vi "I-V扫描.vi"(0 "VISA资源名称":refnum<visa-resource-name>, 1 "nplc":dbl, 3 "时间点(ms)":dbl, 5 "扫描电压(V)":dbl, 9 "电压改变量":dbl, 11 "错误输入":errorcluster, 12 "极限电流(mA)":dbl, 13 "时序优先":bool, 14 "4-wire":bool) -> (4 "VISA资源名称输出":refnum<visa-resource-name>, 6 "扫描数据":dbl[][](array[numeric]), 10 "时间标识":timestamp, 15 "错误输出":errorcluster)   [LabVIEW 2019]
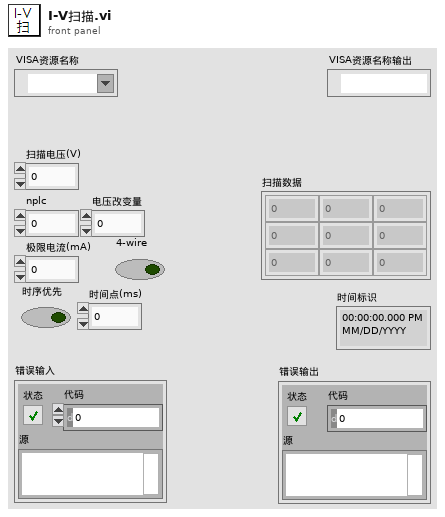
[diagram p1: front panel]
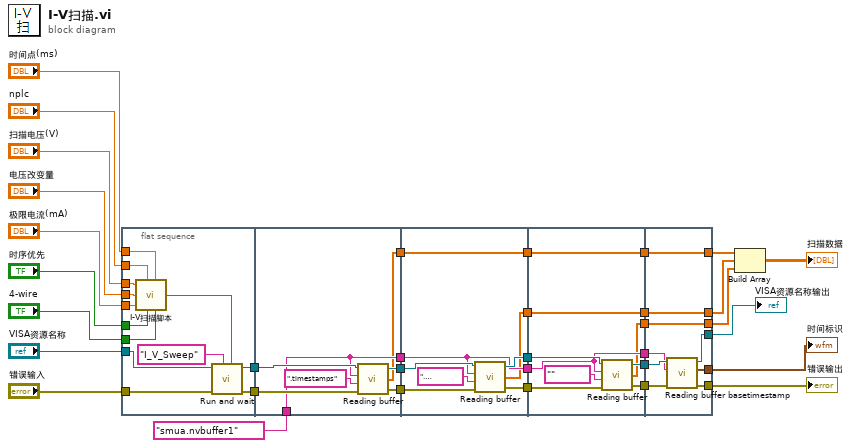
[diagram p0: block diagram]
diagram:
  n1 = flat-sequence {
    tunnel: "错误输入" -> [w46]
    tunnel: "VISA资源名称" -> [w45]
    tunnel: [w44] -> w34
    tunnel: [w43] -> w33
    tunnel: "时间点(ms)" -> [w41]
    tunnel: "时序优先" -> [w40]
    tunnel: "极限电流(mA)" -> [w39]
    tunnel: "电压改变量" -> [w38]
    tunnel: "nplc" -> [w37]
    tunnel: "扫描电压(V)" -> [w36]
    tunnel: "4-wire" -> [w35]
    tunnel: w34 -> [w53]
    tunnel: w33 -> [w52]
    tunnel: [w51] -> w32
    tunnel: [w50] -> w31
    tunnel: [w49] -> w30
    tunnel: "smua.nvbuffer1" ("缓冲区名称") -> [w49]
    tunnel: [w48] -> w29
    tunnel: w32 -> [w61]
    tunnel: w31 -> [w60]
    tunnel: [w59] -> w28
    tunnel: [w58] -> w27
    tunnel: w30 -> [w57]
    tunnel: [w57] -> w26
    tunnel: w29 -> [w56]
    tunnel: [w56] -> w25
    tunnel: [w55] -> w24
    tunnel: w28 -> [w70]
    tunnel: w27 -> [w69]
    tunnel: [w68] -> w23
    tunnel: [w67] -> w22
    tunnel: w26 -> [w66]
    tunnel: [w66] -> w21
    tunnel: w25 -> [w65]
    tunnel: [w65] -> w20
    tunnel: w24 -> [w64]
    tunnel: [w64] -> w19
    tunnel: [w63] -> w18
    tunnel: [w78] -> w14
    tunnel: [w77] -> w15
    tunnel: w23 -> [w80]
    tunnel: w22 -> [w79]
    tunnel: w21 -> [w76]
    tunnel: [w75] -> w12
    tunnel: [w74] -> w10
    tunnel: w20 -> [w74]
    tunnel: w19 -> [w73]
    tunnel: [w73] -> w9
    tunnel: w18 -> [w72]
    tunnel: [w72] -> w8
    frame #0 {
      n2 = call "I-V扫描脚本.vi"("扫描电压(V)"=w36, "nplc"=w37, "电压改变量"=w38, "极限电流(mA)"=w39, "时序优先"=w40, "时间点(ms)"=w41, "4-wire"=w35) -> ("Script"=w42:string)  [unwired: 2 in]
      n3 = call "Run and wait.vi"("Script"=w42, "Script Name"="I_V_Sweep", "错误输入"=w46, "VISA资源名称"=w45) -> ("错误输出"=w44:errorcluster, "VISA资源名称输出"=w43:refnum<visa-resource-name>)  [unwired: 6 in]
    }
    frame #1 {
      n4 = call "Reading buffer.vi"("错误输入"=w53, "Options"=".timestamps", "缓冲区名称"=w49, "VISA资源名称"=w52) -> ("错误输出"=w50:errorcluster, "缓冲区数据"=w48:dbl[], "VISA资源名称输出"=w51:refnum<visa-resource-name>)
    }
    frame #2 {
      n5 = call "Reading buffer.vi"("错误输入"=w60, "Options"=".sourcevalues", "缓冲区名称"=w57, "VISA资源名称"=w61) -> ("错误输出"=w59:errorcluster, "缓冲区数据"=w55:dbl[], "VISA资源名称输出"=w58:refnum<visa-resource-name>)
    }
    frame #3 {
      n6 = call "Reading buffer.vi"("错误输入"=w70, "Options"="", "缓冲区名称"=w66, "VISA资源名称"=w69) -> ("错误输出"=w67:errorcluster, "缓冲区数据"=w63:dbl[], "VISA资源名称输出"=w68:refnum<visa-resource-name>)
    }
    frame #4 {
      n7 = call "Reading buffer basetimestamp.vi"("错误输入"=w79, "缓冲区名称"=w76, "VISA资源名称"=w80) -> ("错误输出"=w78:errorcluster, "时间标识"=w75:timestamp, "VISA资源名称输出"=w77:refnum<visa-resource-name>)  [unwired: 6 in]
    }
  }
  n8 = Build Array(w10, w9, w8) -> (→"扫描数据":dbl[][])
  "VISA资源名称输出" <- w15
  "错误输出" <- w14
  "时间标识" <- w12
